vi "Test_led2_gpio4.vi"(6 "VISA resource name":refnum<visa-resource-name>, 7 "Passed so far?":bool, 8 "error in (no error)":errorcluster, 10 "LED2 ON (y)":bool=TRUE, 11 "Slot":T1) -> (0 "error out":errorcluster, 3 "GPIO4 APx ON?":bool, 4 "VISA resource name out":refnum<visa-resource-name>, 5 "Passed?":bool)   [LabVIEW 2024]
uses:
  AP slots to test.ctl
panel:
  out "GPIO4 AP2 state":string
  out "read buffer AP2":string
  out "GPIO4 AP2 ON?":bool
  out "GPIO4 state":string
  out "read buffer":string
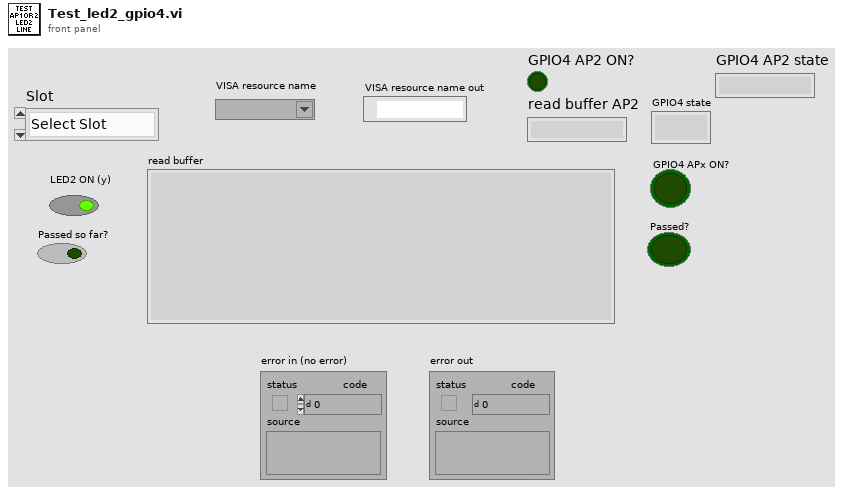
[diagram p1: front panel]
types:
  T1 = typedef "AP slots to test.ctl" = enum16{"Select Slot", "AP1", "AP2", "AP1 and AP2"}
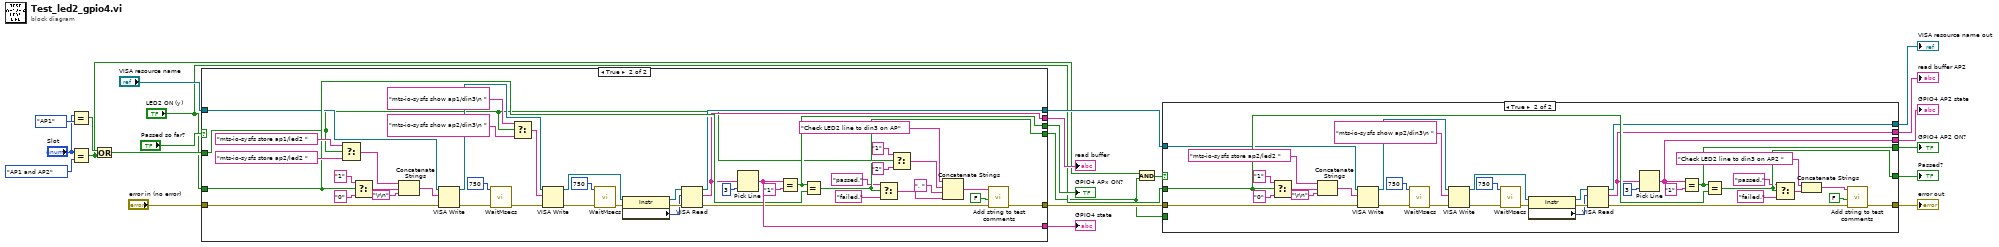
[diagram p0: block diagram]
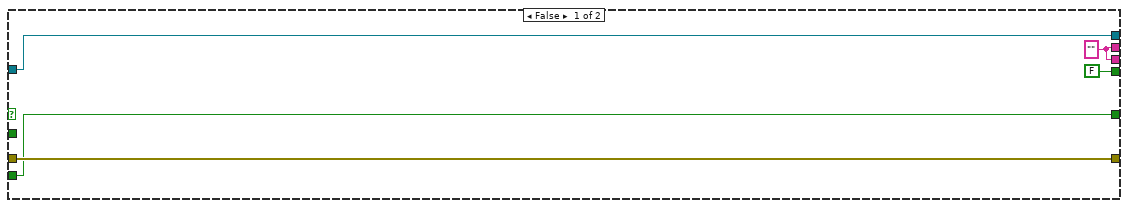
[diagram p2: hidden frame]
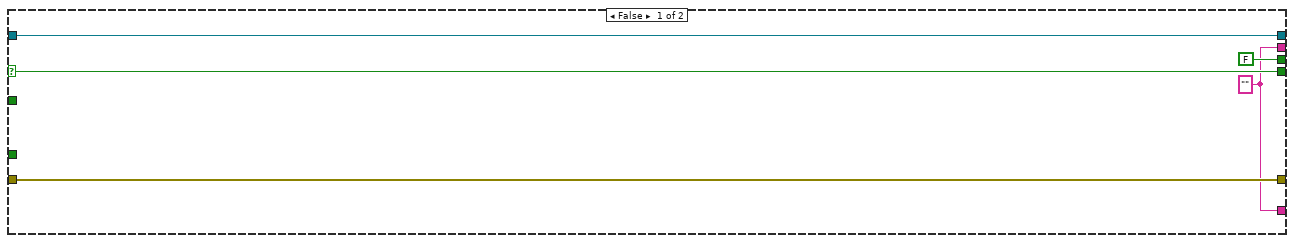
[diagram p3: hidden frame]
diagram:
  n1 = Equal?(x="Slot", y=AP_slots_to_test."AP1") -> (x = y?=w16:bool)
  n2 = Equal?(x="Slot", y=AP_slots_to_test."AP1 and AP2") -> (x = y?=w3:bool)
  n3 = Or(x=w16, y=w3) -> (x .or. y?=w15:bool)
  n4 = case shown="True" "Passed so far?" {
    selector: "Passed so far?" -> [w28 _]
    tunnel: [w25 w41] -> w10
    tunnel: w15 -> [_ w37]
    tunnel: [w24 w56] -> w23
    tunnel: [FALSE w48] -> w22
    tunnel: "LED2 ON (y)" -> [_ w47]
    tunnel: [w28 w34] -> w1
    tunnel: "error in (no error)" -> [w25 w46]
    tunnel: "VISA resource name" -> [w26 w45]
    tunnel: [w26 w44] -> w12
    tunnel: [w24 w42] -> w18
    frame False {
      w24 = "" ("output string")
    }
    frame True {
      n5 = Select(t="mts-io-sysfs store ap1/led2 ", s=w37, f="mts-io-sysfs store ap2/led2 ") -> (s? t:f=w54:string)
      n6 = Select(t="1", s=w47, f="0") -> (s? t:f=w51:string)
      n7 = Concatenate Strings(w54, w51, "\r\n") -> (w50:string)
      n8 = VISA Write(VISA resource name=w45, write buffer=w50, error in (no error)=w46) -> (VISA resource name out=w63:refnum<visa-resource-name>, error out=w67:errorcluster)  [unwired: 1 out]
      n9 = call "WaitMsecs.vi"("error in (no error)"=w67, "Wait Msecs"=u32 750) -> ("error out"=w61:errorcluster)  [unwired: 9 in]
      n10 = Select(t="mts-io-sysfs show ap1/din3\n ", s=w37, f="mts-io-sysfs show ap2/din3\n ") -> (s? t:f=w62:string)
      n11 = VISA Write(VISA resource name=w63, write buffer=w62, error in (no error)=w61) -> (VISA resource name out=w60:refnum<visa-resource-name>, error out=w58:errorcluster)  [unwired: 1 out]
      n12 = call "WaitMsecs.vi"("error in (no error)"=w58, "Wait Msecs"=u32 750) -> ("error out"=w57:errorcluster)  [unwired: 9 in]
      n13 = property class="Instr"(reference=w60, error in=w57) -> (reference out=w72:refnum<visa-resource-name>, error out=w71:errorcluster, "Serial Settings:Number of Bytes at Serial Port"=w70:u32)
      n14 = VISA Read(VISA resource name=w72, byte count=w70, error in (no error)=w71) -> (VISA resource name out=w44:refnum<visa-resource-name>, read buffer=w42:string, error out=w43:errorcluster)  [unwired: 1 out]
      n15 = Pick Line(multi-line string=w42, line index=3) -> (output string=w56:string)  [unwired: 1 in]
      n16 = Equal?(x=w56, y="1") -> (x = y?=w48:bool)
      n17 = Equal?(x=w48, y=w47) -> (x = y?=w34:bool)
      n18 = Select(t="passed.", s=w34, f="failed.") -> (s? t:f=w31:string)
      n19 = Select(t="1", s=w37, f="2") -> (s? t:f=w36:string)
      n20 = Concatenate Strings("Check LED2 line to din3 on AP" ("string"), w36, ", " ("string"), w31) -> (w30:string)
      n21 = call "Add string to test comments.vi"("error in (no error)"=w43, "New Section (y)?"=FALSE, "Comments"=w30) -> ("error out"=w41:errorcluster)  [unwired: 7 in, 1 out]
    }
  }
  "GPIO4 state" <- w23
  "GPIO4 APx ON?" <- w22
  "read buffer" <- w18
  n22 = And(x=w3, y=w1) -> (x .and. y?=w2:bool)
  n23 = case shown="True" w2 {
    tunnel: [w76 w89] -> w9
    tunnel: [w75 w102] -> w4
    tunnel: [FALSE w95] -> w7
    tunnel: "LED2 ON (y)" -> [_ w94]
    tunnel: [w74 w87] -> w8
    tunnel: w10 -> [w76 w81]
    tunnel: w12 -> [w77 w93]
    tunnel: [w77 w92] -> w6
    tunnel: [w75 w90] -> w5
    tunnel: w1 -> [w74 _]
    frame False {
      w75 = "" ("output string")
    }
    frame True {
      n24 = Select(t="1", s=w94, f="0") -> (s? t:f=w98:string)
      n25 = Concatenate Strings("mts-io-sysfs store ap2/led2 ", w98, "\r\n") -> (w97:string)
      n26 = VISA Write(VISA resource name=w93, write buffer=w97, error in (no error)=w81) -> (VISA resource name out=w108:refnum<visa-resource-name>, error out=w110:errorcluster)  [unwired: 1 out]
      n27 = call "WaitMsecs.vi"("error in (no error)"=w110, "Wait Msecs"=u32 750) -> ("error out"=w107:errorcluster)  [unwired: 9 in]
      n28 = VISA Write(VISA resource name=w108, write buffer="mts-io-sysfs show ap2/din3\n ", error in (no error)=w107) -> (VISA resource name out=w106:refnum<visa-resource-name>, error out=w104:errorcluster)  [unwired: 1 out]
      n29 = call "WaitMsecs.vi"("error in (no error)"=w104, "Wait Msecs"=u32 750) -> ("error out"=w103:errorcluster)  [unwired: 9 in]
      n30 = property class="Instr"(reference=w106, error in=w103) -> (reference out=w113:refnum<visa-resource-name>, error out=w112:errorcluster, "Serial Settings:Number of Bytes at Serial Port"=w111:u32)
      n31 = VISA Read(VISA resource name=w113, byte count=w111, error in (no error)=w112) -> (VISA resource name out=w92:refnum<visa-resource-name>, read buffer=w90:string, error out=w91:errorcluster)  [unwired: 1 out]
      n32 = Pick Line(multi-line string=w90, line index=3) -> (output string=w102:string)  [unwired: 1 in]
      n33 = Equal?(x=w102, y="1") -> (x = y?=w95:bool)
      n34 = Equal?(x=w95, y=w94) -> (x = y?=w87:bool)
      n35 = Select(t="passed.", s=w87, f="failed.") -> (s? t:f=w84:string)
      n36 = Concatenate Strings("Check LED2 line to din3 on AP2 " ("string"), w84) -> (w83:string)
      n37 = call "Add string to test comments.vi"("error in (no error)"=w91, "New Section (y)?"=FALSE, "Comments"=w83) -> ("error out"=w89:errorcluster)  [unwired: 7 in, 1 out]
    }
  }
  "error out" <- w9
  "Passed?" <- w8
  "VISA resource name out" <- w6
  "GPIO4 AP2 ON?" <- w7
  "read buffer AP2" <- w5
  "GPIO4 AP2 state" <- w4
